vi "Feature Tracking_distance_calib.vi"(0 "Current Image":T2, 1 "Options":T1={"Level"=6, "Max. Iterations"=20, "Window Size"=50, "Displacement Threshold"=0.01}, 5 "Reference Image":T2, 7 "Location in Pixels":T3(array[cluster]), 11 "error in (no error)":errorcluster) -> (4 "Analysed Image":T2, 6 "Distance Array":dbl[](array[numeric]) caption="DistanceArray", 15 "error out":errorcluster)   [LabVIEW 2020]
doc: "This example shows how to use the Lucas Kanade Pyramid motion estimation VI to track features in a sequence of images in NI Vision. The VI reads the frames from an AVI file and tracks user specified features in the image from frame to frame."
uses:
  <vilib>/vision/Image Controls.llb/IMAQ Image.ctl
  <vilib>/vision/NI_Vision_Development_Module.lvlib
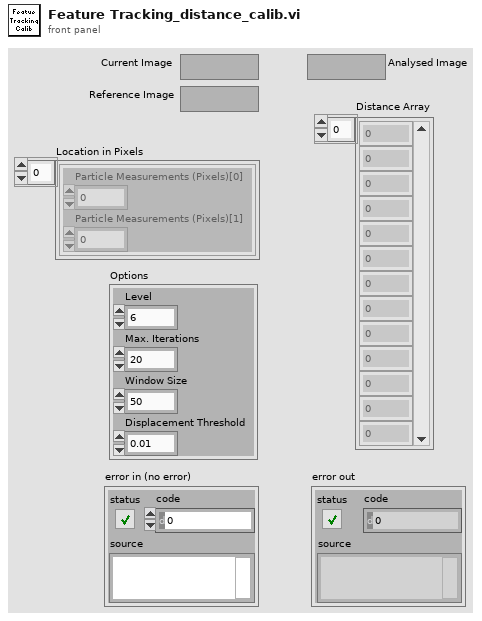
[diagram p1: front panel]
types:
  T1 = cluster{"Level":i32, "Max. Iterations":i32, "Window Size":i32, "Displacement Threshold":dbl}
  T2 = typedef "IMAQ Image.ctl" = refnum<image>
  T3 = cluster{"Particle Measurements (Pixels)[0]":dbl, "Particle Measurements (Pixels)[1]":dbl}[]
  T4 = typedef "Image Type" = u32
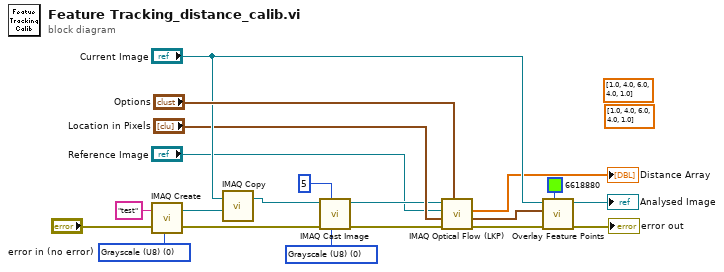
[diagram p0: block diagram]
diagram:
  (unwired) sgl[] [1.0, 4.0, 6.0, 4.0, 1.0] ("Kernel")
  (unwired) sgl[] [1.0, 4.0, 6.0, 4.0, 1.0] ("Kernel")
  w13 = T4 0 items=["Grayscale (U8)", "Grayscale (I16)", "Grayscale (SGL)", "Complex (CSG)", "RGB (U32)", "HSL (U32)", "RGB (U64)", "Grayscale (U16)"] ("Image Type")
  w14 = T4 0 items=["Grayscale (U8)", "Grayscale (I16)", "Grayscale (SGL)", "Complex (CSG)", "RGB (U32)", "HSL (U32)", "RGB (U64)", "Grayscale (U16)"] ("Image Type")
  n1 = call "IMAQ Create"("Image Name"="test", "Image Type"=w13, "error in (no error)"="error in (no error)") -> ("New Image"=w12:T2, "error out"=w7:errorcluster)  [unwired: 2 in]
  n2 = call "IMAQ Copy"("Image Dst"=w12, "Image Src"="Current Image") -> ("Image Dst Out"=w11:T2)  [unwired: 4 in, 1 out]
  n3 = call "IMAQ Cast Image"("Image Type"=w14, "# Shifts"=5, "error in (no error)"=w7, "Image Src"=w11) -> ("error out"=w6:errorcluster, "Image Dst Out"=w4:T2)  [unwired: 6 in]
  n4 = call "IMAQ Optical Flow (LKP)"("Options"="Options", "error in (no error)"=w6, "Feature Points In"="Location in Pixels", "Previous Frame"="Reference Image", "Current Frame"=w4) -> ("error out"=w18:errorcluster, "Feature Points Out"=w19:cluster{"X":sgl, "Y":sgl}[], "Distance Array"=→"Distance Array":dbl[])  [unwired: 1 in, 3 out]
  n5 = call "Overlay Feature Points.vi"("Color"=u32 6618880, "error in"=w18, "Feature Points"=w19, "Image"="Current Image") -> ("error out"=→"error out":errorcluster, "Image Out"=→"Analysed Image":T2)  [unwired: 2 in, 4 out]
